vi "CRYProject Editor PIC Action End.vi"   [LabVIEW 2013]
uses:
  CRYProject Editor Global.vi
  CRYWindow/SubVI/CRYMain Sub Window Global.vi
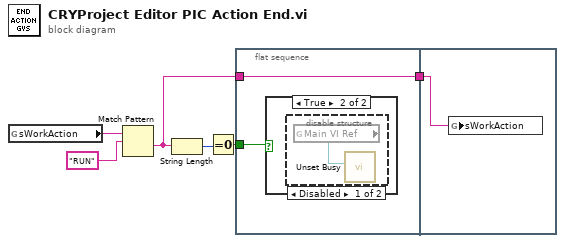
[diagram p0: block diagram]
diagram:
  n1 = global read "CRYProject Editor Global.vi" "sWorkAction"() -> (w6:string)
  n2 = Match Pattern(string=w6, regular expression="RUN" ("sWorkAction")) -> (after substring=w1:string)  [unwired: 1 in, 3 out]
  n3 = String Length(string=w1) -> (length=w4:i32)
  n4 = Equal To 0?(x=w4) -> (x = 0?=w3:bool)
  n5 = flat-sequence {
    tunnel: w3 -> [w8]
    tunnel: [w7] -> w2
    tunnel: w1 -> [w7]
    tunnel: w2 -> [w10]
    frame #0 {
      n6 = case shown="True" w8 {
        frame False {
        }
        frame True {
          n7 = disable-structure shown="Disabled" {
            frame Disabled {
              n8 = global read "CRYMain Sub Window Global.vi" "Main VI Ref"() -> (w9:refnum<vi>)
              n9 = call <vilib>:"Unset Busy.vi"("VI reference (current VI)"=w9) -> ()  [unwired: 10 in, 1 out]
            }
            frame Enabled {
            }
          }
        }
      }
    }
    frame #1 {
      n10 = global write "CRYProject Editor Global.vi" "sWorkAction"(w10) -> ()
    }
  }
